vi "Spartan HTTP Queue Requests.vi"(4 "error in (no error)":errorcluster, 7 "Listener ID":refnum<k5>) -> (0 "error out":errorcluster)   [LabVIEW 2011]
uses:
  Spartan HTTP Server Globals.vi
  ITK EXT/http/http0.llb/HTTP LVHTTP Global.vi
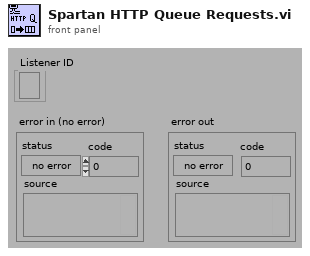
[diagram p1: front panel]
types:
  T1 = typedef "Spartan HTTP Session.ctl" = cluster{"http session":refnum<k1>, "object data":T2, "VI Refnum":refnum<vi>}
  T2 = typedef "HTTP Session Data.ctl" = cluster{"request":string, "time":dbl, "status":i32, "error string":string, "bytes":i32, "env":T3, "content":string, "id":refnum<k5>, "net error":errorcluster}
  T3 = typedef "Keyed Array.ctl" = cluster{"keys":string[], "values":string[]}
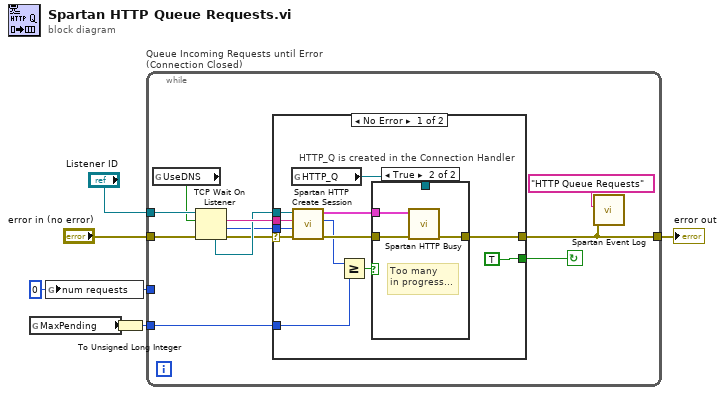
[diagram p0: block diagram]
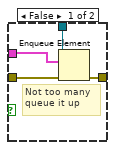
[diagram p2: hidden frame]
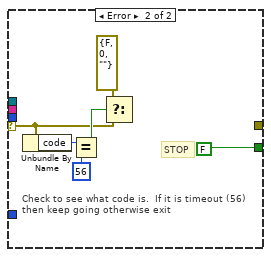
[diagram p3: hidden frame]
diagram:
  w3 = u32 0 ("num requests")
  n1 = global read "HTTP LVHTTP Global.vi" "MaxPending"() -> (w2:i32)
  n2 = global write "Spartan HTTP Server Globals.vi" "num requests"(w3) -> ()
  n3 = To Unsigned Long Integer(number=w2) -> (unsigned 32bit integer=w1:u32)
  n4 = while "Queue Incoming Requests until Error (Connection Closed)" {
    tunnel: "Listener ID" -> [w16]
    tunnel: "error in (no error)" -> [w11]
    tunnel: [w9] -> w5
    tunnel: w3 -> [_]
    tunnel: w1 -> [w7]
    stop <- w8 continue-if-true
    n5 = global read "HTTP LVHTTP Global.vi" "UseDNS"() -> (w13:bool)
    n6 = TCP Wait On Listener(8:w11, 10:w13, 11:w16) -> (0:w12:errorcluster, 1:w14:u16, 2:w17:string, 4:w15:refnum<k5>)  [unwired: 2 out]
    n7 = case shown="No Error" w12 {
      selector: w12 -> [w23 w39]
      tunnel: w17 -> [w25 _]
      tunnel: w15 -> [w26 _]
      tunnel: w14 -> [w24 _]
      tunnel: [w29 _] -> w9
      tunnel: [TRUE FALSE] -> w8
      tunnel: w7 -> [w18 _]
      frame No Error {
        # "HTTP_Q is created in the Connection Handler"
        n8 = global read "Spartan HTTP Server Globals.vi" "HTTP_Q"() -> (w28:refnum<queue>)
        n9 = call "Spartan HTTP Create Session.vi"("error in (no error)"=w23, "remote port"=w24, "address"=w25, "id"=w26) -> ("error out"=w22:errorcluster, "num requests"=w20:u32, "HTTP Data"=w21:T1)  [unwired: 1 out]
        n10 = Greater Or Equal?(x=w20, y=w18) -> (x >= y?=w19:bool)
        n11 = case shown="True" w19 {
          tunnel: w22 -> [w30 w36]
          tunnel: [w33 w35] -> w29
          tunnel: w28 -> [w32 _]
          tunnel: w21 -> [w31 w34]
          frame False {
            # "Not too many\nqueue it up"
            n12 = Enqueue Element(queue=w32, element=w31, error in (no error)=w30) -> (error out=w33:errorcluster)  [unwired: 3 out]
          }
          frame True {
            # "Too many \nin progress..."
            n13 = call "Spartan HTTP Busy.vi"("error in (no error)"=w36, "HTTP Data"=w34) -> ("error out"=w35:errorcluster)  [unwired: 9 out]
          }
        }
      }
      frame Error {
        # "STOP"
        # "Check to see what code is.  If it is timeout (56)\nthen keep going otherwise exit"
        n14 = Unbundle By Name(w39) -> ("code"=w42:i32)
        n15 = Equal?(x=w42, y=56 ("timeout ms (wait forever: -1)")) -> (x = y?=w40:bool)
        n16 = Select(t=errorcluster {"status"=FALSE, "code"=0, "source"=""}, s=w40, f=w39) -> ()  [unwired: 1 out]
      }
    }
    n17 = call "Spartan Event Log.vi"("error in (no error)"=w9, "module (\"\")"="HTTP Queue Requests" ("module (\"\")")) -> ()  [unwired: 3 in, 4 out]
  }
  "error out" <- w5
